vi "Update Controller State.vi"(8 "error in (no error)":errorcluster, 11 "Elevator Controller in":refnum<class "Elevator Controller.lvclass">) -> (0 "error out":errorcluster, 3 "Elevator Controller out":refnum<class "Elevator Controller.lvclass">)   [LabVIEW 2019, in "Elevator Controller Actor.lvlib" / "Elevator Controller.lvclass"]
uses:
  Elevator Controller.lvclass
  Display Console/Display Console/Elevator Direction.ctl
  Display Console/Display Console/Display Console.lvclass
  States -Enum.ctl
  Configuration Database/Configuration Database Messages/Update Displayed Seconds on Timing Msg/Update Displayed Seconds on Timing Msg.lvclass
  Abstract User Console Actor/Abstract User Console Messages/Enable Door Msg/Enable Door Msg.lvclass
  User Console Actor/User Console/Elevator Call.ctl
  User Console Actor/User Console/User Console.lvclass
  User Console Actor/User Console/Floor Selection.ctl
  User Console Actor/User Console/Door Buttons.ctl
  Sensor Interface Actor/Sensor Interface Actor/Sensor Interface.lvclass
  Configuration Database/Configuration Database Actor/Configuration Database.lvclass
  Abstract Display Console Actor/Abstract Display Console Messages/Enable Open Door Msg/Enable Open Door Msg.lvclass
  Abstract User Console Actor/Abstract User Console Messages/Disable all User Console Msg/Disable all User Console Msg.lvclass
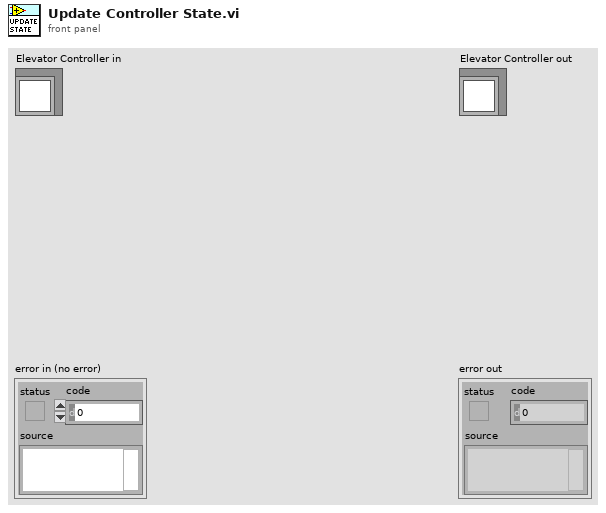
[diagram p1: front panel]
types:
  T1 = typedef "Display Console Actor.lvlib/Display Console.lvclass/Elevator Direction.ctl" = cluster{"Up":bool, "Down":bool}
  T2 = typedef "User Console Actor.lvlib/User Console.lvclass/Door Buttons.ctl" = cluster{"Open Door":bool, "Close Door":bool}
  T3 = typedef "User Console Actor.lvlib/User Console.lvclass/Floor Selection.ctl" = cluster{"Floor4":bool, "Floor 3":bool, "Floor2":bool, "Floor1":bool}
  T4 = typedef "User Console Actor.lvlib/User Console.lvclass/Elevator Call.ctl" = cluster{"Up":bool, "Up 2":bool, "Up 3":bool, "Down":bool, "Down 2":bool, "Down 3":bool}
  T5 = enum8{"Enabled", "Disabled", "Disabled and Grayed Out"}
  T6 = typedef "Elevator Controller Actor.lvlib/Elevator Controller.lvclass/States -Enum.ctl" = enum16{"Initial State", "Start and Move State", "Analysis State", "Continue Travel State", "Open and Close Door Sequence", "Stop at Floor", "No Request remaining", "Emergency Call", "Terminate Process"}
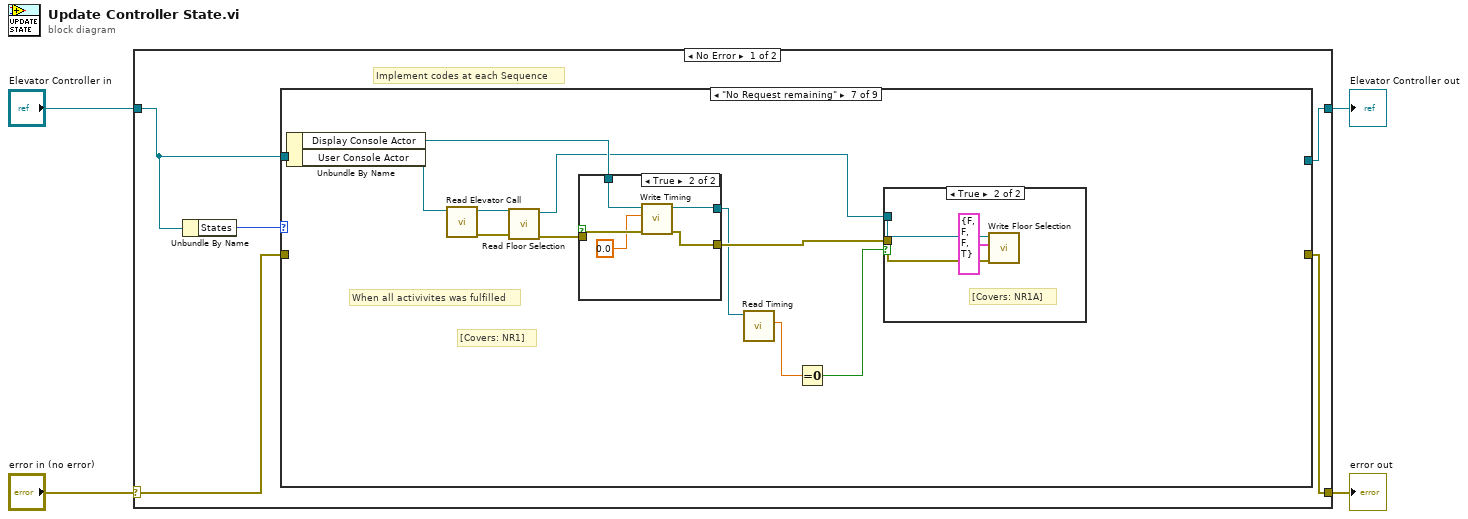
[diagram p0: block diagram]
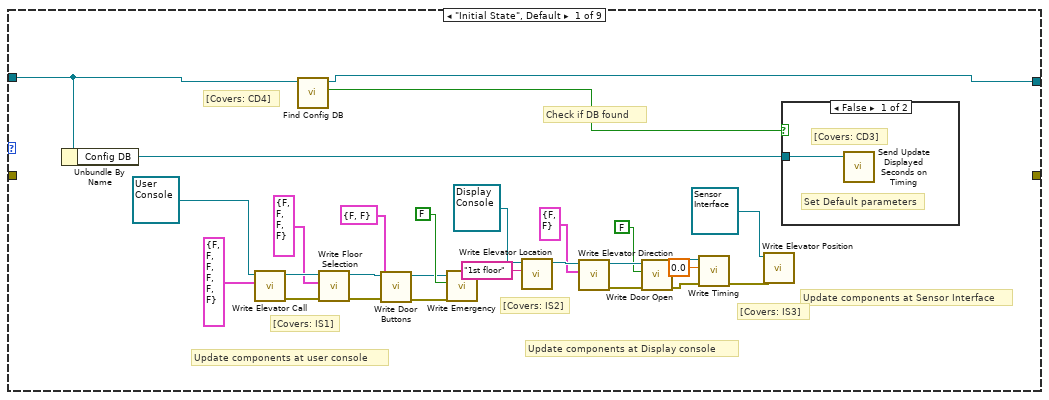
[diagram p2: hidden frame]
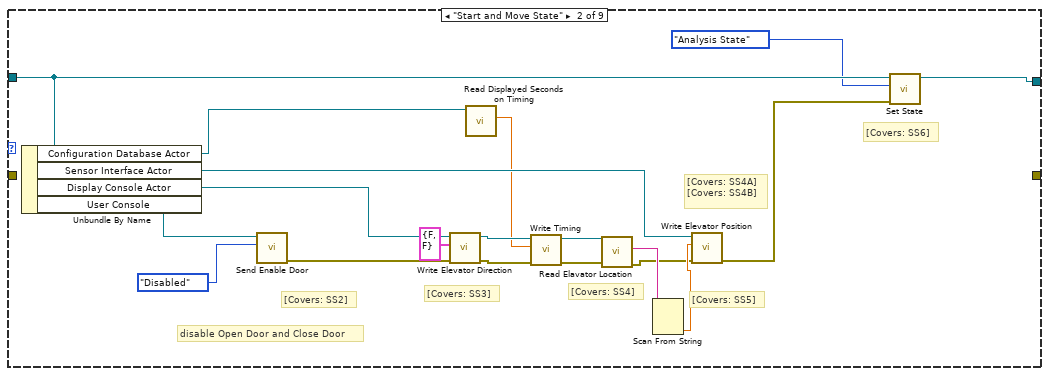
[diagram p4: hidden frame]
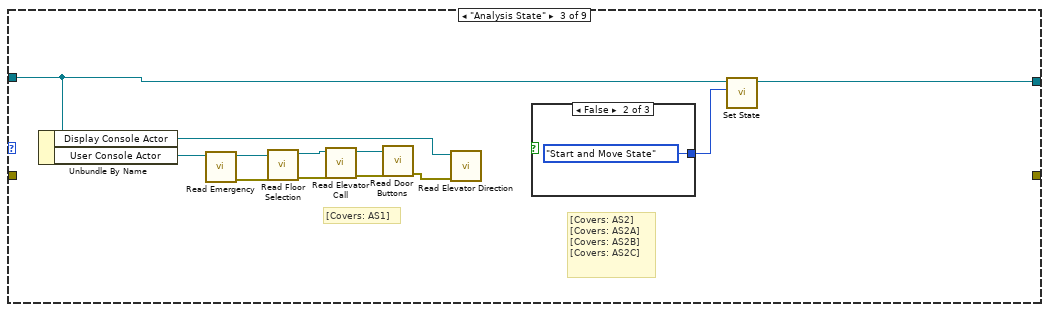
[diagram p5: hidden frame]
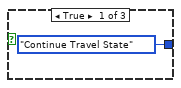
[diagram p6: hidden frame]
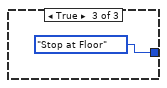
[diagram p7: hidden frame]
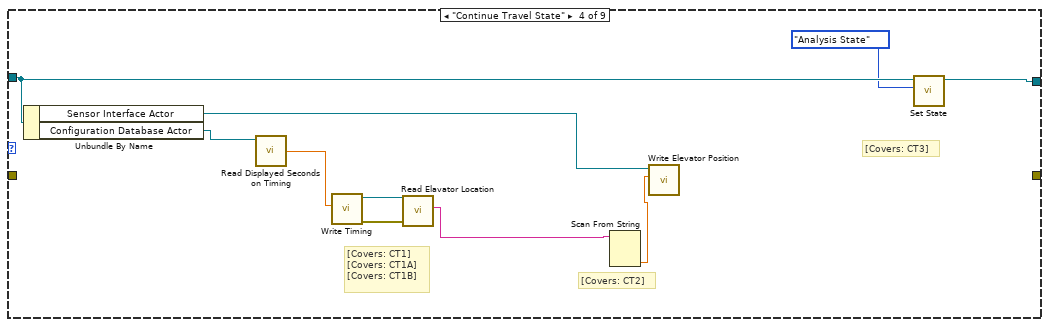
[diagram p8: hidden frame]
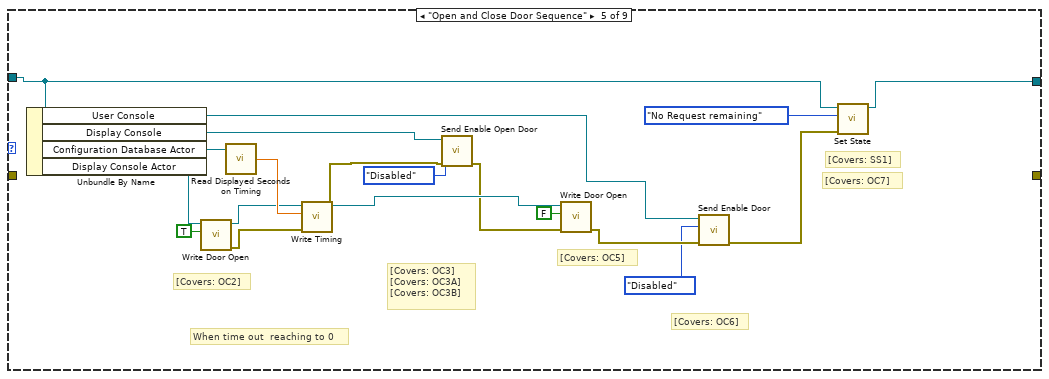
[diagram p9: hidden frame]
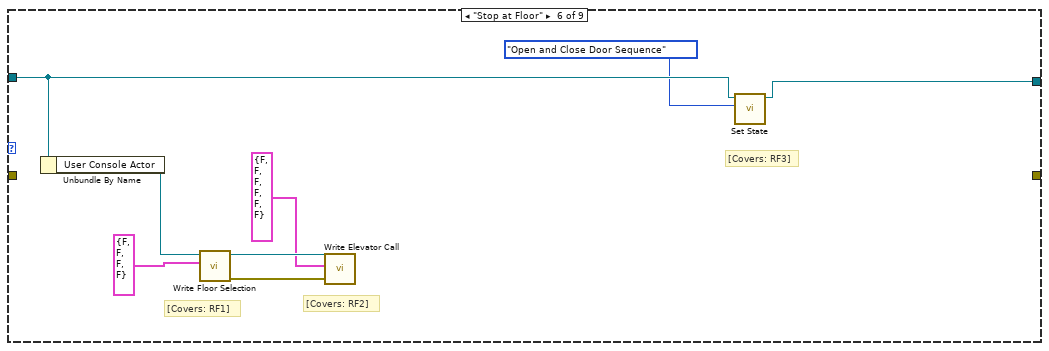
[diagram p10: hidden frame]
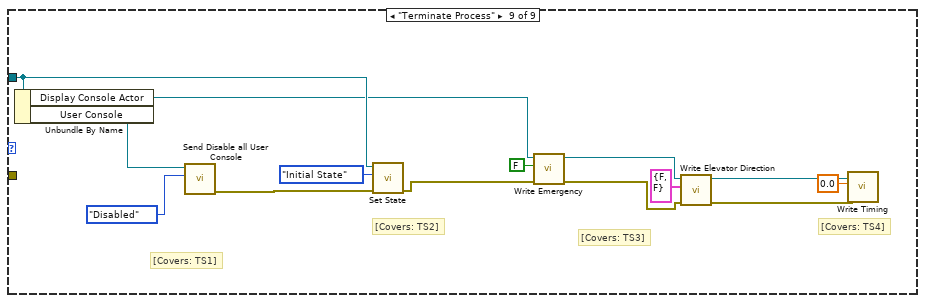
[diagram p14: hidden frame]
diagram:
  n1 = case shown="No Error" "error in (no error)" {
    selector: "error in (no error)" -> [w8 w143]
    tunnel: [w7 w143] -> w3
    tunnel: [w9 w142] -> w1
    tunnel: "Elevator Controller in" -> [w6 w142]
    frame No Error {
      # "Implement codes at each Sequence"
      n2 = Unbundle By Name(w6) -> ("States"=w5:T6)
      n3 = case shown="\"No Request remaining\"" w5 {
        tunnel: w6 -> [w35 w56 w62 w77 w98 w103 w119 _ w139]
        tunnel: [w34 w55 w61 w73 w100 w102 _ _ _] -> w9
        tunnel: w8 -> [_ _ _ _ _ _ _ _ _]
        tunnel: [_ _ _ _ _ _ _ _ _] -> w7
        frame "Initial State", Default {
          # "[Covers: CD4]"
          # "Check if DB found"
          # "Update components at Sensor Interface"
          # "Update components at Display console"
          # "Update components at user console"
          # "[Covers: IS2]"
          # "[Covers: IS1]"
          # "[Covers: IS3]"
          n4 = Unbundle By Name(w35) -> ("Config DB"=w33:refnum<class "Message Enqueuer.lvclass">)
          n5 = call-dynamic "Write Elevator Call.vi"("Elevator Call"=T4 {"Up"=FALSE, "Up 2"=FALSE, "Up 3"=FALSE, "Down"=FALSE, "Down 2"=FALSE, "Down 3"=FALSE}, "User Console in"=refnum<class "User Console.lvclass"> refnum ("User Console Actor.lvlib:User Console.lvclass")) -> ("error out"=w30:errorcluster, "User Console out"=w31:refnum<class "User Console.lvclass">)  [unwired: 8 in]
          n6 = call "Find Config DB.vi"("Elevator Controller in"=w35) -> ("DB Found?"=w36:bool, "Elevator Controller out"=w34:refnum<class "Elevator Controller.lvclass">)  [unwired: 8 in, 1 out]
          n7 = call-dynamic "Write Floor Selection.vi"("error in (no error)"=w30, "Floor Selection"=T3 {"Floor4"=FALSE, "Floor 3"=FALSE, "Floor2"=FALSE, "Floor1"=FALSE}, "User Console in"=w31) -> ("error out"=w27:errorcluster, "User Console out"=w28:refnum<class "User Console.lvclass">)  [unwired: 7 in]
          n8 = call-dynamic "Write Door Buttons.vi"("error in (no error)"=w27, "Door Buttons"=T2 {"Open Door"=FALSE, "Close Door"=FALSE}, "User Console in"=w28) -> ("error out"=w24:errorcluster, "User Console out"=w23:refnum<class "User Console.lvclass">)  [unwired: 7 in]
          n9 = call-dynamic "Write Emergency.vi"("error in (no error)"=w24, "Emergency Button"=FALSE, "User Console in"=w23) -> ()  [unwired: 7 in, 2 out]
          n10 = call-dynamic "Write Elevator Location.vi"("Elevator Position"="1st floor", "Display Console in"=refnum<class "Display Console.lvclass"> refnum ("Display Console Actor.lvlib:Display Console.lvclass")) -> ("Display Console out"=w19:refnum<class "Display Console.lvclass">)  [unwired: 8 in, 1 out]
          n11 = call-dynamic "Write Elevator Direction.vi"("Elevator Direction"=T1 {"Up"=FALSE, "Down"=FALSE}, "Display Console in"=w19) -> ("error out"=w16:errorcluster, "Display Console out"=w17:refnum<class "Display Console.lvclass">)  [unwired: 8 in]
          n12 = call-dynamic "Write Door Open.vi"("error in (no error)"=w16, "Door Open"=FALSE, "Display Console in"=w17) -> ("error out"=w13:errorcluster, "Display Console out"=w14:refnum<class "Display Console.lvclass">)  [unwired: 7 in]
          n13 = call-dynamic "Write Timing.vi"("error in (no error)"=w13, "timing"=0.0, "Display Console in"=w14) -> ("error out"=w10:errorcluster)  [unwired: 7 in, 1 out]
          n14 = call-dynamic "Write Elevator Position.vi"("error in (no error)"=w10, "Sensor Interface in"=refnum<class "Sensor Interface.lvclass"> refnum ("Sensor Interface Actor.lvlib:Sensor Interface.lvclass")) -> ()  [unwired: 8 in, 2 out]
          n15 = case shown="False" w36 {
            tunnel: w33 -> [w37 _]
            frame False {
              # "[Covers: CD3]"
              # "Set Default parameters"
              n16 = call "Send Update Displayed Seconds on Timing.vi"("Message Enqueuer"=w37) -> ()  [unwired: 9 in, 2 out]
            }
            frame True {
            }
          }
        }
        frame "Start and Move State" {
          # "[Covers: SS5]"
          # "[Covers: SS4A] \n[Covers: SS4B]"
          # "[Covers: SS4]"
          # "[Covers: SS3]"
          # "[Covers: SS2]"
          # "disable Open Door and Close Door"
          # "[Covers: SS6]"
          n17 = Unbundle By Name(w56) -> ("Configuration Database Actor"=w39:refnum<class "Configuration Database.lvclass">, "Sensor Interface Actor"=w46:refnum<class "Sensor Interface.lvclass">, "Display Console Actor"=w50:refnum<class "Display Console.lvclass">, "User Console"=w53:refnum<class "Message Enqueuer.lvclass">)
          n18 = call "Send Enable Door.vi"("Disabled"=T5."Disabled", "Message Enqueuer"=w53) -> ("error out"=w51:errorcluster)  [unwired: 8 in, 1 out]
          n19 = call-dynamic "Write Elevator Direction.vi"("error in (no error)"=w51, "Elevator Direction"=T1 {"Up"=FALSE, "Down"=FALSE}, "Display Console in"=w50) -> ("error out"=w48:errorcluster, "Display Console out"=w47:refnum<class "Display Console.lvclass">)  [unwired: 7 in]
          n20 = call "Read Displayed Seconds on Timing.vi"("Configuration Database in"=w39) -> ("Time(Sec)"=w38:dbl)  [unwired: 8 in, 2 out]
          n21 = call-dynamic "Write Timing.vi"("error in (no error)"=w48, "timing"=w38, "Display Console in"=w47) -> ("error out"=w41:errorcluster, "Display Console out"=w45:refnum<class "Display Console.lvclass">)  [unwired: 7 in]
          n22 = call-dynamic "Read Elavator Location.vi"("error in (no error)"=w41, "Display Console in"=w45) -> ("error out"=w40:errorcluster, "Elevator Position"=w44:string)  [unwired: 7 in, 1 out]
          n23 = Scan From String(input string=w44) -> (output 1=w43:dbl)  [unwired: 4 in, 3 out]
          n24 = call-dynamic "Write Elevator Position.vi"("error in (no error)"=w40, "Elevator Position"=w43, "Sensor Interface in"=w46) -> ("error out"=w42:errorcluster)  [unwired: 7 in, 1 out]
          n25 = call "Set State.vi"("error in (no error)"=w42, "States"=States_-Enum."Analysis State", "Elevator Controller in"=w56) -> ("Elevator Controller out"=w55:refnum<class "Elevator Controller.lvclass">)  [unwired: 7 in, 1 out]
        }
        frame "Analysis State" {
          # "[Covers: AS1]"
          # "[Covers: AS2] \n[Covers: AS2A] \n[Covers: AS2B] \n[Covers: AS2C]"
          n26 = Unbundle By Name(w62) -> ("Display Console Actor"=w64:refnum<class "Display Console.lvclass">, "User Console Actor"=w68:refnum<class "User Console.lvclass">)
          n27 = call-dynamic "Read Emergency.vi"("User Console in"=w68) -> ("error out"=w59:errorcluster, "User Console out"=w67:refnum<class "User Console.lvclass">)  [unwired: 8 in, 1 out]
          n28 = call-dynamic "Read Floor Selection.vi"("error in (no error)"=w59, "User Console in"=w67) -> ("error out"=w58:errorcluster, "User Console out"=w66:refnum<class "User Console.lvclass">)  [unwired: 7 in, 1 out]
          n29 = call-dynamic "Read Elevator Call.vi"("error in (no error)"=w58, "User Console in"=w66) -> ("error out"=w57:errorcluster, "User Console out"=w65:refnum<class "User Console.lvclass">)  [unwired: 7 in, 1 out]
          n30 = call-dynamic "Read Door Buttons.vi"("error in (no error)"=w57, "User Console in"=w65) -> ("error out"=w63:errorcluster)  [unwired: 7 in, 2 out]
          n31 = call-dynamic "Read Elevator Direction.vi"("error in (no error)"=w63, "Display Console in"=w64) -> ()  [unwired: 7 in, 3 out]
          n32 = case shown="\"Change Direction\"" {
            selector: _ -> [_ _ _]
            tunnel: [States_-Enum."Continue Travel State" ("States") States_-Enum."Start and Move State" ("States") States_-Enum."Stop at Floor" ("States")] -> w60
            frame True {
            }
            frame False {
            }
            frame True {
            }
          }
          n33 = call "Set State.vi"("States"=w60, "Elevator Controller in"=w62) -> ("Elevator Controller out"=w61:refnum<class "Elevator Controller.lvclass">)  [unwired: 8 in, 1 out]
        }
        frame "Continue Travel State" {
          # "[Covers: CT2]"
          # "[Covers: CT1]\n[Covers: CT1A] \n[Covers: CT1B]"
          # "[Covers: CT3]"
          n34 = Unbundle By Name(w77) -> ("Sensor Interface Actor"=w74:refnum<class "Sensor Interface.lvclass">, "Configuration Database Actor"=w78:refnum<class "Configuration Database.lvclass">)
          n35 = call "Read Displayed Seconds on Timing.vi"("Configuration Database in"=w78) -> ("Time(Sec)"=w79:dbl)  [unwired: 8 in, 2 out]
          n36 = call-dynamic "Write Timing.vi"("timing"=w79) -> ("error out"=w80:errorcluster, "Display Console out"=w81:refnum<class "Display Console.lvclass">)  [unwired: 9 in]
          n37 = call-dynamic "Read Elavator Location.vi"("error in (no error)"=w80, "Display Console in"=w81) -> ("Elevator Position"=w75:string)  [unwired: 7 in, 2 out]
          n38 = Scan From String(input string=w75) -> (output 1=w76:dbl)  [unwired: 4 in, 3 out]
          n39 = call-dynamic "Write Elevator Position.vi"("Elevator Position"=w76, "Sensor Interface in"=w74) -> ()  [unwired: 8 in, 2 out]
          n40 = call "Set State.vi"("States"=States_-Enum."Analysis State", "Elevator Controller in"=w77) -> ("Elevator Controller out"=w73:refnum<class "Elevator Controller.lvclass">)  [unwired: 8 in, 1 out]
        }
        frame "Open and Close Door Sequence" {
          # "[Covers: OC6]"
          # "[Covers: OC5]"
          # "When time out  reaching to 0"
          # "[Covers: OC3] \n[Covers: OC3A] \n[Covers: OC3B]"
          # "[Covers: OC7]"
          # "[Covers: OC2]"
          # "[Covers: SS1]"
          n41 = Unbundle By Name(w98) -> ("User Console"=w84:refnum<class "Message Enqueuer.lvclass">, "Display Console"=w91:refnum<class "Message Enqueuer.lvclass">, "Configuration Database Actor"=w94:refnum<class "Configuration Database.lvclass">, "Display Console Actor"=w97:refnum<class "Display Console.lvclass">)
          n42 = call-dynamic "Write Door Open.vi"("Door Open"=TRUE, "Display Console in"=w97) -> ("error out"=w93:errorcluster, "Display Console out"=w92:refnum<class "Display Console.lvclass">)  [unwired: 8 in]
          n43 = call "Read Displayed Seconds on Timing.vi"("Configuration Database in"=w94) -> ("Time(Sec)"=w95:dbl)  [unwired: 8 in, 2 out]
          n44 = call-dynamic "Write Timing.vi"("error in (no error)"=w93, "timing"=w95, "Display Console in"=w92) -> ("error out"=w89:errorcluster, "Display Console out"=w88:refnum<class "Display Console.lvclass">)  [unwired: 7 in]
          n45 = call "Send Enable Open Door.vi"("error in (no error)"=w89, "Disabled"=T5."Disabled", "Message Enqueuer"=w91) -> ("error out"=w87:errorcluster)  [unwired: 7 in, 1 out]
          n46 = call-dynamic "Write Door Open.vi"("error in (no error)"=w87, "Door Open"=FALSE, "Display Console in"=w88) -> ("error out"=w85:errorcluster)  [unwired: 7 in, 1 out]
          n47 = call "Send Enable Door.vi"("error in (no error)"=w85, "Disabled"=T5."Disabled", "Message Enqueuer"=w84) -> ("error out"=w82:errorcluster)  [unwired: 7 in, 1 out]
          n48 = call "Set State.vi"("error in (no error)"=w82, "States"=States_-Enum."No Request remaining", "Elevator Controller in"=w98) -> ("Elevator Controller out"=w100:refnum<class "Elevator Controller.lvclass">)  [unwired: 7 in, 1 out]
        }
        frame "Stop at Floor" {
          # "[Covers: RF3]"
          # "[Covers: RF2]"
          # "[Covers: RF1]"
          n49 = Unbundle By Name(w103) -> ("User Console Actor"=w108:refnum<class "User Console.lvclass">)
          n50 = call-dynamic "Write Floor Selection.vi"("Floor Selection"=T3 {"Floor4"=FALSE, "Floor 3"=FALSE, "Floor2"=FALSE, "Floor1"=FALSE}, "User Console in"=w108) -> ("error out"=w105:errorcluster, "User Console out"=w106:refnum<class "User Console.lvclass">)  [unwired: 8 in]
          n51 = call-dynamic "Write Elevator Call.vi"("error in (no error)"=w105, "Elevator Call"=T4 {"Up"=FALSE, "Up 2"=FALSE, "Up 3"=FALSE, "Down"=FALSE, "Down 2"=FALSE, "Down 3"=FALSE}, "User Console in"=w106) -> ()  [unwired: 7 in, 2 out]
          n52 = call "Set State.vi"("States"=States_-Enum."Open and Close Door Sequence", "Elevator Controller in"=w103) -> ("Elevator Controller out"=w102:refnum<class "Elevator Controller.lvclass">)  [unwired: 8 in, 1 out]
        }
        frame "No Request remaining" {
          # "When all activivites was fulfilled"
          # "[Covers: NR1]"
          n53 = Unbundle By Name(w119) -> ("Display Console Actor"=w116:refnum<class "Display Console.lvclass">, "User Console Actor"=w109:refnum<class "User Console.lvclass">)
          n54 = call-dynamic "Read Elevator Call.vi"("User Console in"=w109) -> ("error out"=w117:errorcluster, "User Console out"=w118:refnum<class "User Console.lvclass">)  [unwired: 8 in, 1 out]
          n55 = call-dynamic "Read Floor Selection.vi"("error in (no error)"=w117, "User Console in"=w118) -> ("error out"=w115:errorcluster, "User Console out"=w110:refnum<class "User Console.lvclass">)  [unwired: 7 in, 1 out]
          n56 = case shown="True" {
            selector: _ -> [_ _]
            tunnel: w116 -> [_ w127]
            tunnel: w115 -> [_ w126]
            tunnel: [_ w124] -> w114
            tunnel: [_ w123] -> w113
            frame False {
            }
            frame True {
              n57 = call-dynamic "Write Timing.vi"("error in (no error)"=w126, "timing"=0.0, "Display Console in"=w127) -> ("error out"=w124:errorcluster, "Display Console out"=w123:refnum<class "Display Console.lvclass">)  [unwired: 7 in]
            }
          }
          n58 = call-dynamic "Read Timing.vi"("Display Console in"=w113) -> ("timing"=w112:dbl)  [unwired: 8 in, 2 out]
          n59 = Equal To 0?(x=w112) -> (x = 0?=w111:bool)
          n60 = case shown="True" w111 {
            tunnel: w114 -> [_ w122]
            tunnel: w110 -> [_ w121]
            frame False {
              # "[Covers: NR1B]"
            }
            frame True {
              # "[Covers: NR1A]"
              n61 = call-dynamic "Write Floor Selection.vi"("error in (no error)"=w122, "Floor Selection"=T3 {"Floor4"=FALSE, "Floor 3"=FALSE, "Floor2"=FALSE, "Floor1"=TRUE}, "User Console in"=w121) -> ()  [unwired: 7 in, 2 out]
            }
          }
        }
        frame "Emergency Call" {
        }
        frame "Terminate Process" {
          # "[Covers: TS4]"
          # "[Covers: TS3]"
          # "[Covers: TS2]"
          # "[Covers: TS1]"
          n62 = Unbundle By Name(w139) -> ("Display Console Actor"=w134:refnum<class "Display Console.lvclass">, "User Console"=w140:refnum<class "Message Enqueuer.lvclass">)
          n63 = call "Send Disable all User Console.vi"("Disabled"=T5."Disabled", "Message Enqueuer"=w140) -> ("error out"=w138:errorcluster)  [unwired: 8 in, 1 out]
          n64 = call "Set State.vi"("error in (no error)"=w138, "States"=States_-Enum."Initial State", "Elevator Controller in"=w139) -> ("error out"=w131:errorcluster)  [unwired: 7 in, 1 out]
          n65 = call-dynamic "Write Emergency.vi"("error in (no error)"=w131, "Emergency"=FALSE, "Display Console in"=w134) -> ("error out"=w132:errorcluster, "Display Console out"=w133:refnum<class "Display Console.lvclass">)  [unwired: 7 in]
          n66 = call-dynamic "Write Elevator Direction.vi"("error in (no error)"=w132, "Elevator Direction"=T1 {"Up"=FALSE, "Down"=FALSE}, "Display Console in"=w133) -> ("error out"=w128:errorcluster, "Display Console out"=w130:refnum<class "Display Console.lvclass">)  [unwired: 7 in]
          n67 = call-dynamic "Write Timing.vi"("error in (no error)"=w128, "timing"=0.0, "Display Console in"=w130) -> ()  [unwired: 7 in, 2 out]
        }
      }
    }
    frame Error {
    }
  }
  "error out" <- w3
  "Elevator Controller out" <- w1
